vi "FuncImg-Extract selected ROIs data.vi"(8 "error in (no error)":errorcluster) -> (0 "error out":errorcluster, 1 "ROI numbers":i32[](array[numeric]), 2 "Data for ticked ROI":T1, 3 "Total number of points":i32, 4 "X-axis max/min":cluster{"X-axis max":dbl, "X-axis min":dbl}, 5 "Points in each trial":i32)   [LabVIEW 2013]
uses:
  xcontrol/Interface VIs/Interface typedefs/Interface-Data array.ctl
  xcontrol/Interface VIs/Interface typedefs/Interface-Data format definition.ctl
  xcontrol/Typedefs/Xctl-XY data type definition.ctl
  xcontrol/Typedefs/Xctrl-ROI type enum.ctl
  Experiment header interface/Typedefs/Header parameters cluster-Zstack.ctl
  Typedefs/Frame Size.ctl
  Global variables/gl_Functional Imaging-Global variables.vi
  xcontrol/XGrapher.xctl
panel:
  # "<--- Timeline data already decimated\n          for memory efficiency."
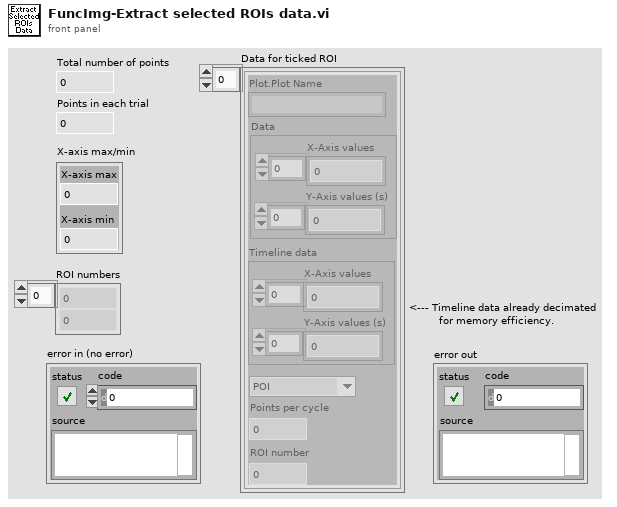
[diagram p1: front panel]
types:
  T1 = typedef "Interface-Data array.ctl" = T2[]
  T2 = typedef "Interface-Data format definition.ctl" = cluster{"Plot.Plot Name":string, "Data":T3, "Timeline data":T3, "Type":T4, "Points per cycle":u16, "ROI number":u16}
  T3 = typedef "XGrapher.xctl/Xctl-XY data type definition.ctl" = cluster{"X-Axis values":sgl[], "Y-Axis values (s)":i32[]}
  T4 = typedef "Xctrl-ROI type enum.ctl" = enum16{"POI", "Mini-scan", "Group"}
  T5 = typedef "Header parameters cluster-Zstack.ctl" = cluster{"Number of POI":u16, "Number of Miniscans":u16, "Number of Trials":u16, "Number of Cycles ":u16, "# Averaged Frames":u16, "Laser power (%)":u8, "Pockels":dbl, "Acquisition Length (sec)":dbl, "Fill time (us)":dbl, "DwellTime (us)":dbl, "Miniscan Dwell time per pixel (us)":dbl, "PMT 1":dbl, "PMT 2":dbl, "Back Apperture":dbl, "Zoom":dbl, "Number of Pixels in Miniscan":u16, "Frame Size":T6, "Field of View":dbl, "X centre":dbl, "Y centre":dbl, "AOL Z":dbl}
  T6 = typedef "Frame Size.ctl" = u16
  T7 = cluster{"Channel A?":bool, "Cycle length (us)":dbl, "[Pixels in ROI]":i32[], "Z-Stack Header data":T5, "[ROI Time (us)]":dbl[], "Path out":path, "Version index":i32}
  T8 = typedef "Functional Imging UI Refs.ctl" = cluster{"Menu ref":refnum<k9>, "Image control":refnum<vi>, "VI ref":refnum<vi>, "XGrapher":refnum<vi>, "Smoothing":refnum<vi>, "POI Averaging":refnum<vi>, "Normalize":refnum<vi>, "POI data points in each trial":refnum<vi>, "Channel":refnum<vi>, "Experiment data folder path":refnum<vi>, "[ROI vis]":refnum<vi>, "[Groups] visbl":T9, "Group Name":refnum<vi>, "POI index":refnum<vi>, "Trial No.":refnum<vi>, "Intensity Zoom":refnum<vi>, "Trial Cursor Enabled":refnum<vi>, "Number of Trials (ind 1)":refnum<vi>, "Number of Trials (ind 2)":refnum<vi>, "MiniScans Available":refnum<vi>, "POI Available":refnum<vi>, "Defer graph updates":refnum<vi>, "Waveform selector":refnum<vi>, "#of selected POI":refnum<vi>, "#of selected MiniScans":refnum<vi>, "#of selected groups":refnum<vi>, "Max Z-Projection":refnum<vi>, "Z-Plane Selector":refnum<vi>, "Index of miniscan point to visualise":refnum<vi>, "ROI vis. mode":refnum<vi>, "Total # of points":refnum<vi>, "Index of group clicked on":refnum<vi>, "Pane 1":refnum<vi>, "Pane 2":refnum<vi>, "Pane 3":refnum<vi>, "Pane 4":refnum<vi>, "Pane 5":refnum<vi>, "Pane 6":refnum<vi>, "Deselect all ROI":refnum<vi>, "Deselect all groups":refnum<vi>}
  T9 = typedef "Groups array referecne.ctl" = refnum<vi>
  T10 = typedef "ROI selector array.ctl" = T11[]
  T11 = typedef "Interface-ROI selection cluster.ctl" = cluster{"ROI number":i32, "ROI ID":T12, "Visibility":bool}
  T12 = typedef "ROI ID Enum.ctl" = enum16{"Point", "MiniScan", "Comp. MiniScan", "Rectangle", "Comp. volume", "Arb. plane point"}
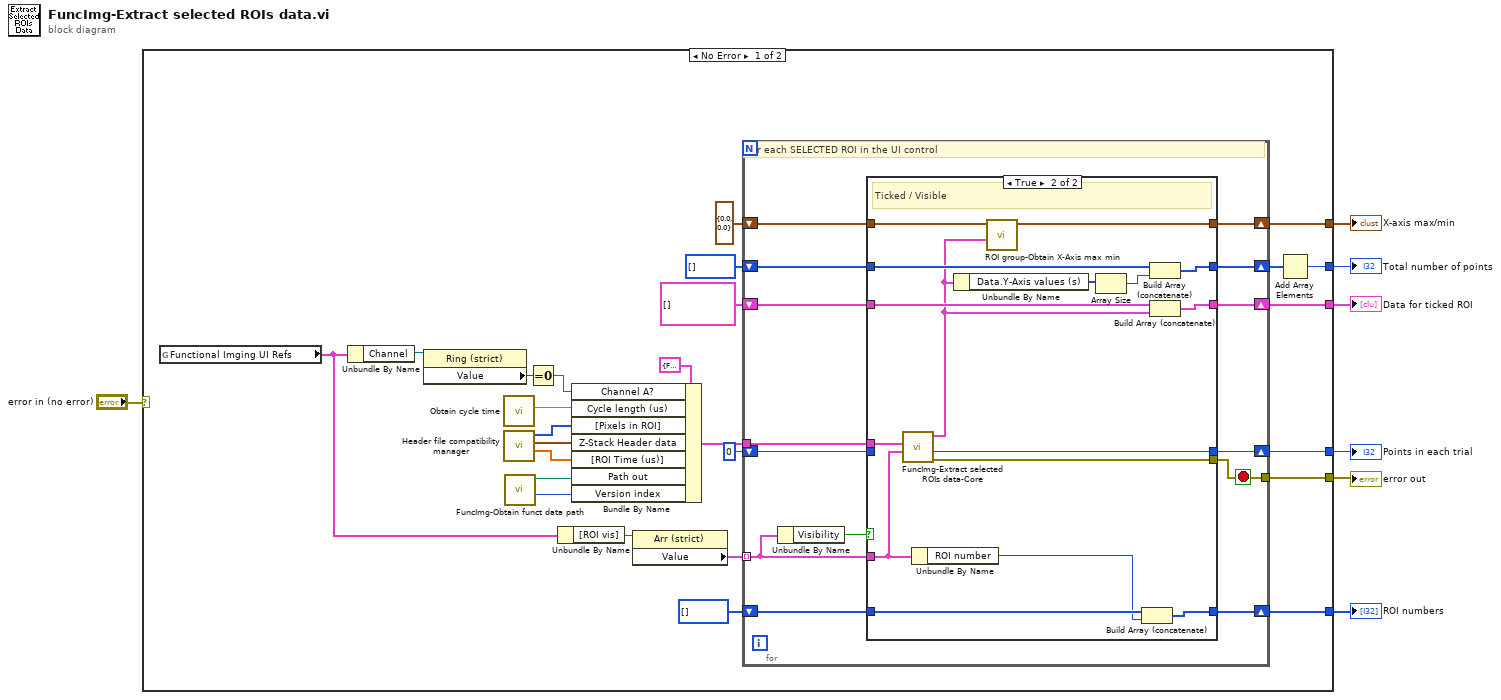
[diagram p0: block diagram]
diagram:
  n1 = case shown="No Error" "error in (no error)" {
    selector: "error in (no error)" -> [_ w69]
    tunnel: [w33 _] -> w7
    tunnel: [w30 _] -> w6
    tunnel: [w25 _] -> w5
    tunnel: [w8 _] -> w4
    tunnel: [w10 _] -> w3
    tunnel: [w9 w69] -> w2
    frame No Error {
      n2 = global read "gl_Functional Imaging-Global variables.vi" "Functional Imging UI Refs"() -> (w13:T8)
      n3 = Unbundle By Name(w13) -> ("Channel"=w14:refnum<vi>)
      n4 = property on="Property Node" class="Ring (strict)"(reference=w14) -> ("Value"=w22:u16)  [unwired: 1 in, 2 out]
      n5 = call "Obtain cycle time.vi"() -> ("Funct Acq cycle length (us)"=w15:dbl)  [unwired: 10 in, 1 out]
      n6 = call "Header file compatibility manager.vi"() -> ("[ROI Time (us)]"=w19:dbl[], "Z-Stack Header data"=w18:T5, "[Pixels in ROI]"=w17:i32[])  [unwired: 8 in, 1 out]
      n7 = call "FuncImg-Obtain funct data path.vi"() -> ("Version index (-1 = latest version)"=w21:i32, "Functional data folder path"=w20:path)  [unwired: 7 in, 3 out]
      n8 = Equal To 0?(x=w22) -> (x = 0?=w23:bool)
      n9 = Unbundle By Name(w13) -> ("[ROI vis]"=w29:refnum<vi>)
      n10 = Bundle By Name(cluster=T7 {"Channel A?"=FALSE, "Cycle length (us)"=0.0, "[Pixels in ROI]"=[], "Z-Stack Header data"={"Number of POI"=0, "Number of Miniscans"=0, "Number of Trials"=0, "Number of Cycles "=0, "# Averaged Frames"=0, "Laser power (%)"=0, "Pockels"=0.0, "Acquisition Length (sec)"=0.0, "Fill time (us)"=0.0, "DwellTime (us)"=0.0, "Miniscan Dwell time per pixel (us)"=0.0, "PMT 1"=0.0, "PMT 2"=0.0, "Back Apperture"=0.0, "Zoom"=0.0, "Number of Pixels in Miniscan"=0, "Frame Size"=200, "Field of View"=0.0, "X centre"=0.0, "Y centre"=0.0, "AOL Z"=0.0}, "[ROI Time (us)]"=[], "Path out"=path "", "Version index"=0} ("Cluster"), "Channel A?"=w23, "Cycle length (us)"=w15, "[Pixels in ROI]"=w17, "Z-Stack Header data"=w18, "[ROI Time (us)]"=w19, "Path out"=w20, "Version index"=w21) -> (w12:T7)
      n11 = property on="Property Node" class="Arr (strict)"(reference=w29) -> ("Value"=w31:T10)  [unwired: 1 in, 2 out]
      n12 = for {
        tunnel: w31 -> [w43] mode=indexing
        shift-right: [w46] -> w8
        shift-left: T1 [] ("element") -> [w39]
        shift-right: [w45] -> w32
        shift-left: i32[] [] -> [w40]
        shift-right: [w44] -> w10
        shift-left: cluster{dbl, dbl} {0.0, 0.0} ("Max min out") -> [w41]
        shift-right: [w47] -> w30
        shift-left: 0 -> [w36]
        shift-right: [w37] -> w25
        shift-left: i32[] [] ("ROI indexes") -> [w38]
        tunnel: w12 -> [w35]
        tunnel: [w34] -> w9
        stop <- w34 stop-if-true
        # "For each SELECTED ROI in the UI control"
        n13 = Unbundle By Name(w43) -> ("Visibility"=w42:bool)
        n14 = case shown="True" w42 {
          tunnel: [w49 w59] -> w47
          tunnel: [w50 w68] -> w46
          tunnel: [w51 w67] -> w45
          tunnel: [w52 w56] -> w44
          tunnel: w43 -> [_ w58]
          tunnel: w41 -> [w52 w55]
          tunnel: w40 -> [w51 w66]
          tunnel: w39 -> [w50 w65]
          tunnel: w38 -> [w48 w64]
          tunnel: [w48 w63] -> w37
          tunnel: w36 -> [w49 _]
          tunnel: w35 -> [_ w62]
          tunnel: [_ w53] -> w34
          frame False {
            # "Unticked / Not visible"
          }
          frame True {
            # "Ticked / Visible"
            n15 = call "FuncImg-Extract selected ROIs data-Core.vi"("System Cluster"=w58, "Input cluster"=w62) -> ("error IO"=w53:errorcluster, "Points per trial"=w59:i32, "Interface-Data format definition"=w54:T2)  [unwired: 7 in]
            n16 = Unbundle By Name(w58) -> ("ROI number"=w57:i32)
            n17 = Unbundle By Name(w54) -> ("Data.Y-Axis values (s)"=w61:i32[])
            n18 = call "ROI group-Obtain X-Axis max min.vi"("ROI group data"=w54, "Max min-shift in"=w55) -> ("Max min out"=w56:cluster{dbl, dbl})  [unwired: 9 in]
            n19 = Array Size(array=w61) -> (size(s)=w60:i32)
            n20 = Build Array (concatenate)(w64, w57) -> (w63:i32[])
            n21 = Build Array (concatenate)(w66, w60) -> (w67:i32[])
            n22 = Build Array (concatenate)(w65, w54) -> (w68:T1)
          }
        }
      }
      n23 = Add Array Elements(numeric array=w32) -> (sum=w33:i32)
    }
    frame Error {
    }
  }
  "Total number of points" <- w7
  "Data for ticked ROI" <- w4
  "Points in each trial" <- w6
  "X-axis max/min" <- w3
  "ROI numbers" <- w5
  "error out" <- w2
